vi "attoDRYexample lv16.vi"() -> ()   [LabVIEW 2016]
uses:
  <userlib>/attoDRYLib/attoDRYLib.lvlib
panel:
  out "4K plate/magnet temperature":dbl
  out "Temperature Controlling":bool
  out "ControllingTemperature out":i32
  in  "COM Port":refnum<visa-resource-name>
  in  "Start/Stop Measurement":bool
  out "User Temperature":dbl
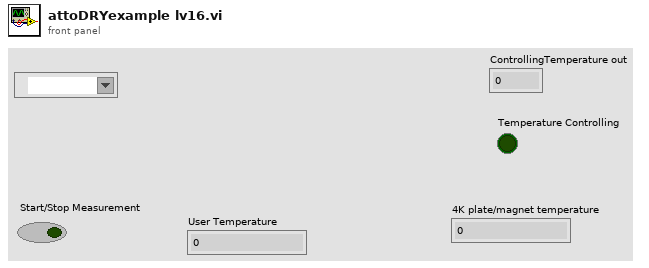
[diagram p1: front panel]
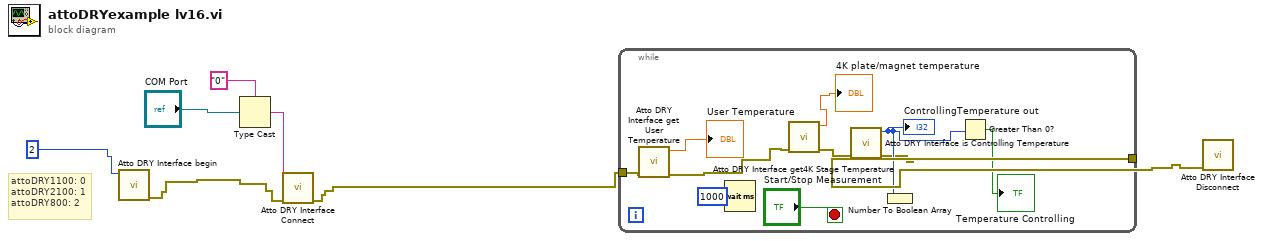
[diagram p0: block diagram]
diagram:
  # "attoDRY1100: 0\nattoDRY2100: 1\nattoDRY800: 2"
  n1 = call <userlib>:"Atto DRY Interface begin.vi"("Device"=u16 2) -> ("error out"=w3:errorcluster)  [unwired: 9 in, 1 out]
  n2 = Type Cast(type="0", x="COM Port") -> (*(type *) &x=w2:string)
  n3 = call <userlib>:"Atto DRY Interface Connect.vi"("error in (no error)"=w3, "COMPort"=w2) -> ("error out"=w4:errorcluster)  [unwired: 7 in, 2 out]
  n4 = while {
    tunnel: w4 -> [w12]
    tunnel: [w13] -> w1
    stop <- "Start/Stop Measurement" stop-if-true
    n5 = call <userlib>:"Atto DRY Interface get User Temperature.vi"("error in (no error)"=w12) -> ("error out"=w10:errorcluster, "Temperature out"=→"User Temperature":sgl)  [unwired: 8 in, 1 out]
    n6 = Wait (ms)(milliseconds to wait=1000) -> ()  [unwired: 1 out]
    n7 = call <userlib>:"Atto DRY Interface get4K Stage Temperature.vi"("error in (no error)"=w10) -> ("error out"=w9:errorcluster, "_4KStageTemperatureK out"=→"4K plate/magnet temperature":sgl)  [unwired: 8 in, 1 out]
    n8 = call <userlib>:"Atto DRY Interface is Controlling Temperature.vi"("error in (no error)"=w9) -> ("error out"=w13:errorcluster, "ControllingTemperature out"=w14:i32)  [unwired: 8 in, 1 out]
    "ControllingTemperature out" <- w14
    n9 = Number To Boolean Array(number=w14) -> ()  [unwired: 1 out]
    n10 = Greater Than 0?(x=w14) -> (x > 0?=→"Temperature Controlling":bool)
  }
  n11 = call <userlib>:"Atto DRY Interface Disconnect.vi"("error in (no error)"=w1) -> ()  [unwired: 9 in, 2 out]
